vi "mead_and_deviation.vi"(2 "insieme":dbl[][](array[numeric])) -> (0 "Dev":dbl[](array[numeric]), 1 "Media":dbl[](array[numeric]))   [LabVIEW 2021, in "CALIBRATION.lvlib"]
uses:
  <vilib>/Analysis/baseanly.llb/Mean (DBL).vi
  CALIBRATION.lvlib
  <vilib>/Analysis/NI_AALBase.lvlib
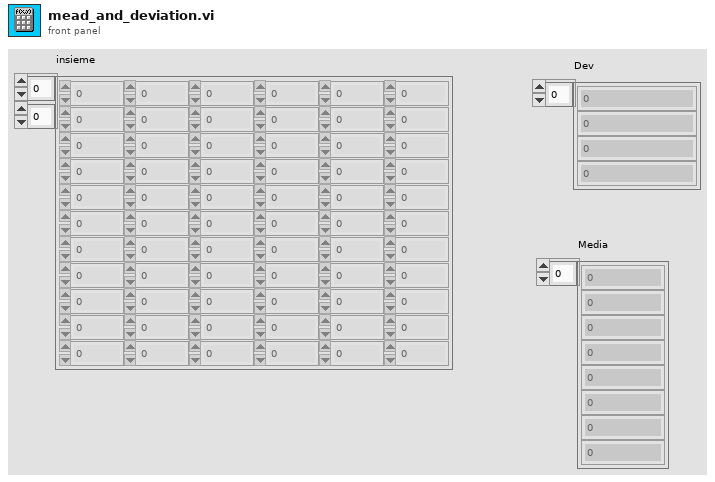
[diagram p1: front panel]
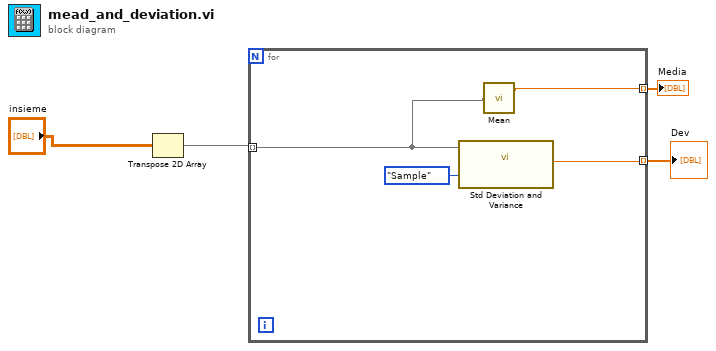
[diagram p0: block diagram]
diagram:
  n1 = Transpose 2D Array(2D array="insieme") -> (transposed array=w2:dbl[][])
  n2 = for {
    tunnel: [w5] -> w3 mode=indexing
    tunnel: [w8] -> w4 mode=indexing
    tunnel: w2 -> [w6] mode=indexing
    # "SALITA/DISCESA 1"
    n3 = call <vilib>:"Std Deviation and Variance.vi"("X"=w6, "Weighting (Sample)"=enum16{"Sample", "Population"}."Sample") -> ("standard deviation"=w5:dbl)  [unwired: 2 out]
    n4 = call-poly <vilib>:"Mean.vi"("X"=w6) -> ("mean"=w8:dbl)  [unwired: 1 out]
  }
  "Media" <- w4
  "Dev" <- w3
